vi "CreateTableDC.vi"(8 "error in (no error)":errorcluster, 10 "Name of Table":string, 11 "DataCollector in":refnum<class "DataCollector.lvclass">) -> (0 "error out":errorcluster, 3 "DataCollector out":refnum<class "DataCollector.lvclass">)   [LabVIEW 2017, in "DataCollector.lvclass"]
uses:
  DataCollector.lvclass
  DataCollector.lvclass/DataCollector.ctl
  <vilib>/drjdpowell/SQLite Library/SQL Connection/Execute SQL.vi
  <vilib>/drjdpowell/SQLite Library/SQL Connection/Execute SQL (Single Integer).vi
  <vilib>/drjdpowell/SQLite Library/SQLite.lvlib
  <vilib>/drjdpowell/SQLite Library/SQL Connection/Connection.lvclass
panel:
  out "concatenated string":string
  out "Result Set":string[][](table) caption="Result Set (from first statement with results)"
  out "Column Names":string[](array[string])
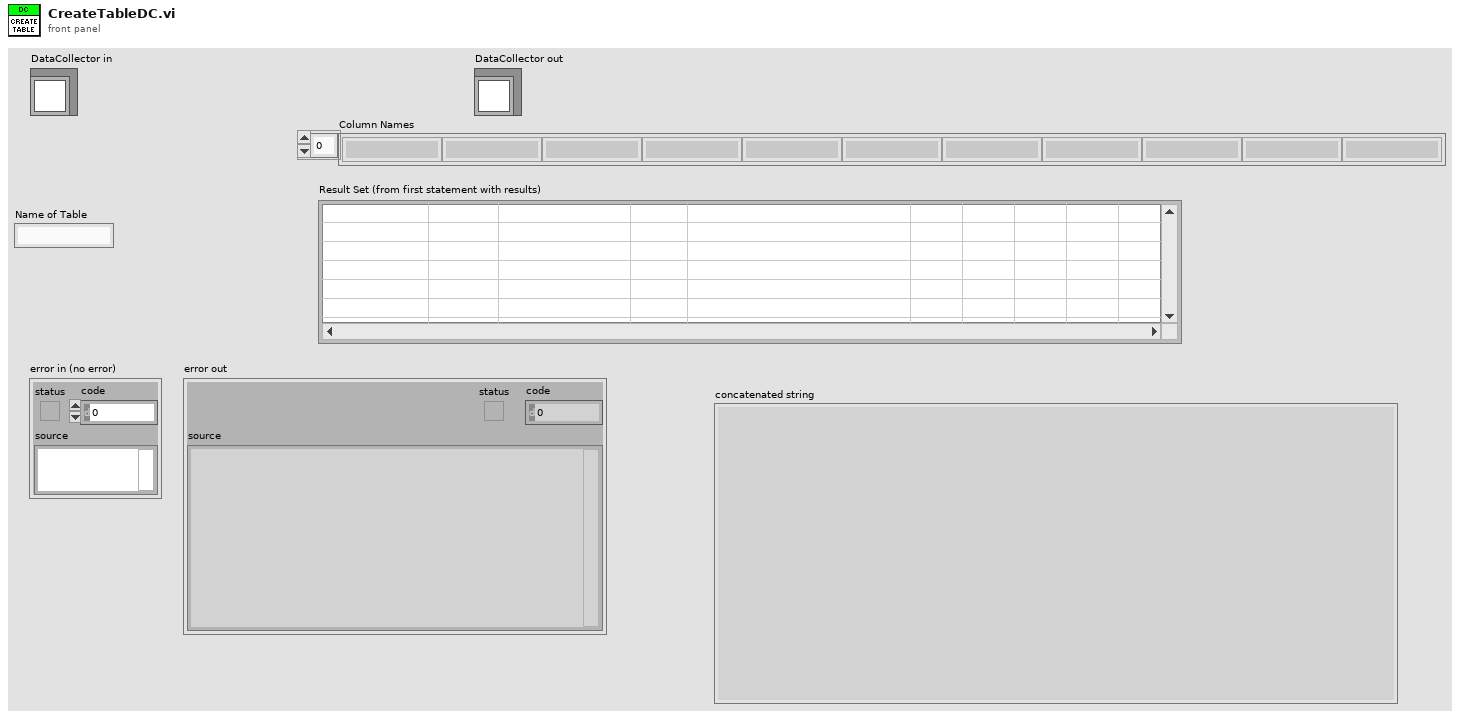
[diagram p1: front panel]
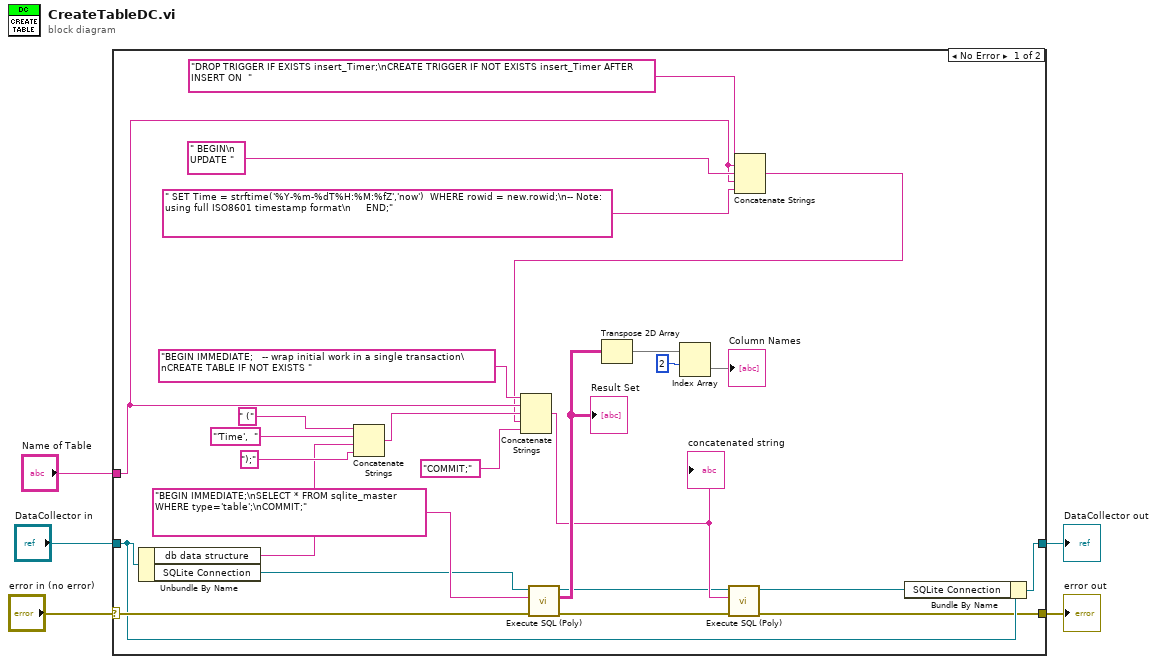
[diagram p0: block diagram]
diagram:
  n1 = case shown="No Error" "error in (no error)" {
    selector: "error in (no error)" -> [w28 w33]
    tunnel: [w16 w33] -> w5
    tunnel: [w25 w32] -> w4
    tunnel: "DataCollector in" -> [w23 w32]
    tunnel: "Name of Table" -> [w10 _]
    frame No Error {
      n2 = Unbundle By Name(w23) -> ("db data structure"=w7:string, "SQLite Connection"=w24:refnum<class "Connection.lvclass">)
      n3 = Concatenate Strings(" (" ("string"), "'Time',  " ("string"), w7, ");" ("string")) -> (w15:string)
      n4 = call-poly <vilib>:"Execute SQL (Poly).vi"("error in (no error)"=w28, "SQL"="BEGIN IMMEDIATE;\nSELECT * FROM sqlite_master WHERE type='table';\nCOMMIT;" ("String"), "SQLite Connection in"=w24) -> ("error out"=w17:errorcluster, "Result Set"=w29:string[][], "SQLite Connection out"=w18:refnum<class "Connection.lvclass">)  [unwired: 5 in, 1 out]
      "Result Set" <- w29
      n5 = Transpose 2D Array(2D array=w29) -> (transposed array=w31:string[][])
      n6 = Index Array(array=w31, index (row)=2 ("Index")) -> (element=→"Column Names":string[])  [unwired: 1 in]
      n7 = Concatenate Strings("DROP TRIGGER IF EXISTS insert_Timer;\nCREATE TRIGGER IF NOT EXISTS insert_Timer AFTER  INSERT ON  ", w10, " BEGIN\n UPDATE ", w10, " SET Time = strftime('%Y-%m-%dT%H:%M:%fZ','now')  WHERE rowid = new.rowid;\n-- Note: using full ISO8601 timestamp format\n     END;") -> (w8:string)
      n8 = Concatenate Strings("BEGIN IMMEDIATE;   -- wrap initial work in a single transaction\nCREATE TABLE IF NOT EXISTS ", w10, w15, w8, "COMMIT;" ("string")) -> (w20:string)
      "concatenated string" <- w20
      n9 = call-poly <vilib>:"Execute SQL (Poly).vi"("error in (no error)"=w17, "SQL"=w20, "SQLite Connection in"=w18) -> ("error out"=w16:errorcluster, "SQLite Connection out"=w19:refnum<class "Connection.lvclass">)  [unwired: 6 in, 1 out]
      n10 = Bundle By Name(cluster=w23, "SQLite Connection"=w19) -> (w25:refnum<class "DataCollector.lvclass">)
    }
    frame Error {
    }
  }
  "error out" <- w5
  "DataCollector out" <- w4
